vi "Convert Frequencies.vi"(4 "Resonance Frequency (MHz)":dbl[unit]=100000000.0, 5 "Number of Intervals":u32, 6 "Start Frequency (MHz)":dbl[unit], 7 "Stop Frequency (MHz)":dbl[unit]) -> (0 "Start Frequency (Number)":dbl, 1 "Frequency Increment (Number)":dbl, 2 "Number of Intervals (Out)":u32, 3 "Frequency Interval":dbl[unit])   [LabVIEW 2009]
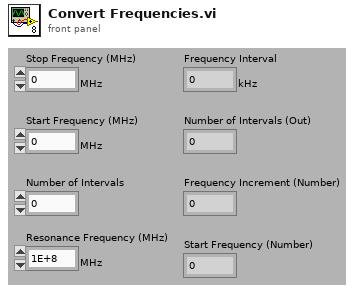
[diagram p1: front panel]
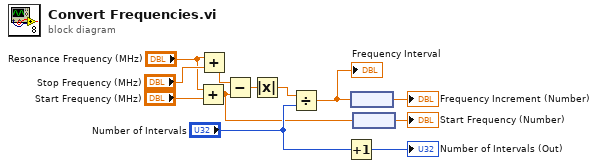
[diagram p0: block diagram]
diagram:
  n1 = Add(x="Resonance Frequency (MHz)", y="Start Frequency (MHz)") -> (x+y=w1:dbl[unit])
  n2 = Add(x="Resonance Frequency (MHz)", y="Stop Frequency (MHz)") -> (x+y=w4:dbl[unit])
  n3 = Subtract(x=w4, y=w1) -> (x-y=w12:dbl[unit])
  n4 = Absolute Value(x=w12) -> (abs(x)=w11:dbl[unit])
  n5 = Divide(x=w11, y="Number of Intervals") -> (x/y=w9:dbl[unit])
  "Frequency Interval" <- w9
  n6 = Increment(x="Number of Intervals") -> (x+1=→"Number of Intervals (Out)":u32)
  n7 = node(w9) -> (→"Frequency Increment (Number)":dbl)
  n8 = node(w1) -> (→"Start Frequency (Number)":dbl)
